vi "compute_adv.vi"(1 "param":T1={"Srated"=25000.0, "eta [pu]"=0.98, "model"={"in-states"={"v1"=0.0, "v2"=0.0, "SoC"=0.0}, "output"={"V"=0.0, "Zeq"=0.0, "Eeq"=0.0}}} {"model"."output"."Eeq" format="%#.6g"; "model"."output"."Zeq" format="%#.6g"; "eta [pu]" format="%#_13g"}, 2 "SoC_T":dbl, 3 "Meas":T2 {"Ud" format="%#.2f"; "P" format="%#.2f"; "Q" format="%#.2f"}) -> (0 "json-adv":string)   [LabVIEW 2021]
uses:
  General purpose/MEAS.ctl
  General purpose/agent-variables.ctl
  General purpose/BA-ADV.ctl
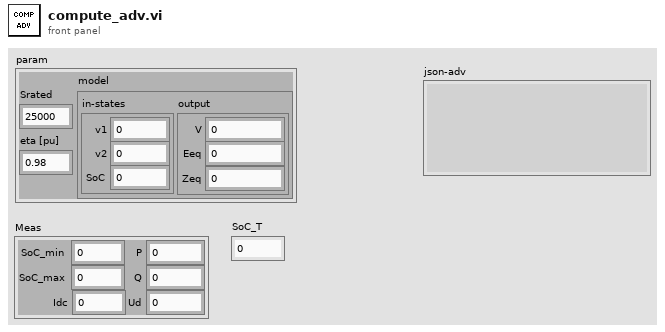
[diagram p1: front panel]
types:
  T1 = typedef "agent-variables.ctl" = cluster{"Srated":dbl, "eta [pu]":dbl, "model":cluster{"in-states":cluster{"v1":dbl, "v2":dbl, "SoC":dbl}, "output":cluster{"V":dbl, "Zeq":dbl, "Eeq":dbl}}}
  T2 = typedef "MEAS.ctl" = cluster{"P":dbl, "Q":dbl, "SoC_max":dbl, "SoC_min":dbl, "Ud":dbl, "Idc":dbl}
  T3 = typedef "BA-ADV.ctl" = cluster{"Pimp":dbl, "Qimp":dbl, "Pmin":dbl, "Pmax":dbl, "Srated":dbl, "coeffP":dbl, "coeffPsquared":dbl, "SoE":dbl, "coeffQsquared":dbl, "coeffQ":dbl}
  T4 = typedef "cost-function.ctl" = cluster{"coeffPsquared":dbl, "coeffP":dbl, "coeffQsquared":dbl, "coeffQ":dbl}
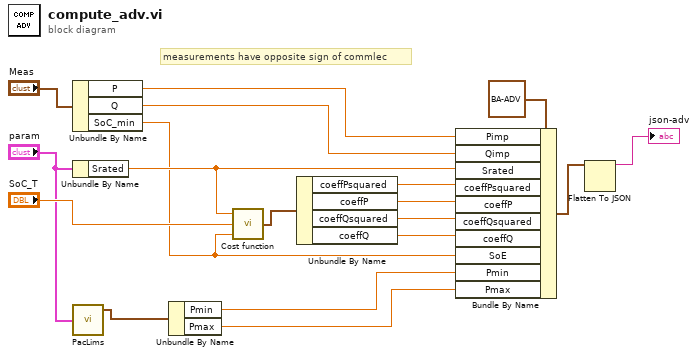
[diagram p0: block diagram]
diagram:
  # "measurements have opposite sign of commlec"
  n1 = Unbundle By Name("Meas") -> ("P"=w18:dbl, "Q"=w16:dbl, "SoC_min"=w13:dbl)
  n2 = Unbundle By Name("param") -> ("Srated"=w15:dbl)
  n3 = call "PacLims.vi"("param (in)"="param") -> ("PacLims"=w14:cluster{"Pmax":dbl, "Pmin":dbl})  [unwired: 2 out]
  n4 = Unbundle By Name(w14) -> ("Pmin"=w9:dbl, "Pmax"=w8:dbl)
  n5 = call "Cost function.vi"("SoC"=w13, "SoC_T"="SoC_T", "Srated"=w15) -> ("cost-function"=w5:T4)
  n6 = Unbundle By Name(w5) -> ("coeffPsquared"=w4:dbl, "coeffP"=w3:dbl, "coeffQsquared"=w2:dbl, "coeffQ"=w1:dbl)
  n7 = Bundle By Name(cluster=T3 {"Pimp"=0.0, "Qimp"=0.0, "Pmin"=0.0, "Pmax"=0.0, "Srated"=0.0, "coeffP"=0.0, "coeffPsquared"=0.0, "SoE"=0.0, "coeffQsquared"=0.0, "coeffQ"=0.0} ("ADV"), "Pimp"=w18, "Qimp"=w16, "Srated"=w15, "coeffPsquared"=w4, "coeffP"=w3, "coeffQsquared"=w2, "coeffQ"=w1, "SoE"=w13, "Pmin"=w9, "Pmax"=w8) -> (w11:T3)
  n8 = Flatten To JSON(anything=w11) -> (JSON string=→"json-adv":string)  [unwired: 2 in, 1 out]
